vi "update display current.vi"(8 "error in (no error)":errorcluster, 11 "focus in":refnum<class "focus.lvclass">) -> (0 "error out":errorcluster, 3 "focus out":refnum<class "focus.lvclass">)   [LabVIEW 2012, in "focus.lvclass"]
uses:
  focus.lvclass
  focus.lvclass/focus.ctl
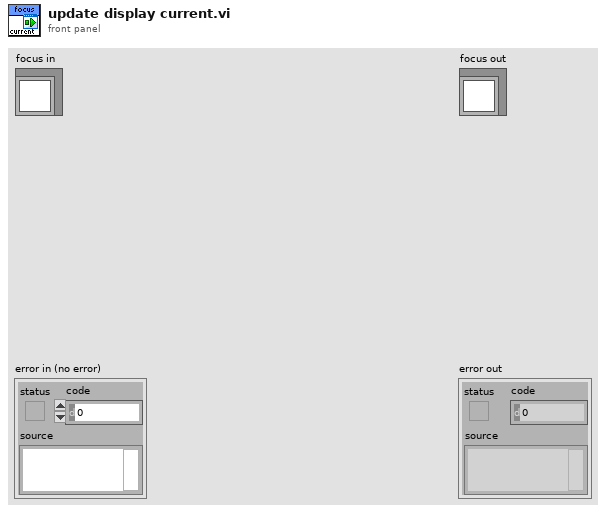
[diagram p1: front panel]
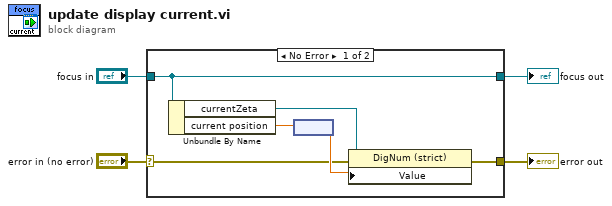
[diagram p0: block diagram]
diagram:
  n1 = case shown="No Error" "error in (no error)" {
    selector: "error in (no error)" -> [w6 w12]
    tunnel: [w5 w12] -> w3
    tunnel: [w10 w11] -> w1
    tunnel: "focus in" -> [w10 w11]
    frame No Error {
      n2 = Unbundle By Name(w10) -> ("currentZeta"=w8:refnum<vi>, "current position"=w7:dbl)
      n3 = node(w7) -> (w9:dbl[unit])
      n4 = property class="DigNum (strict)"(reference=w8, error in=w6, "Value"=w9) -> (error out=w5:errorcluster)  [unwired: 1 out]
    }
    frame Error {
    }
  }
  "error out" <- w3
  "focus out" <- w1
